vi "VelocityRamp_r0.vi"(10 "Current Velocity (RPS)":dbl, 11 "Input Velocity (RPS)":dbl) -> (3 "Output Velocity (RPS)":dbl)   [LabVIEW 2015]
panel:
  in  "Step Delay (ms)":u32
  out "Waveform Chart":dbl(graph)
  in  "Step Size":dbl format="%#_13g"
  in  "Threshold":dbl format="%#_13g"
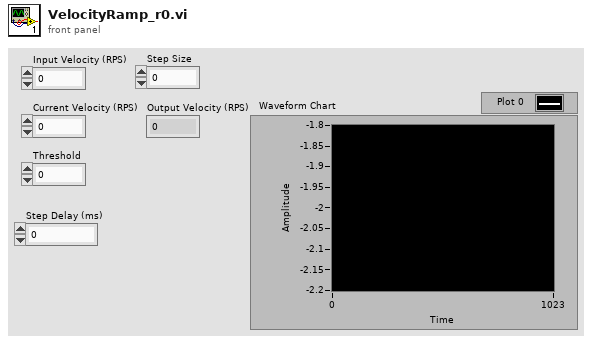
[diagram p1: front panel]
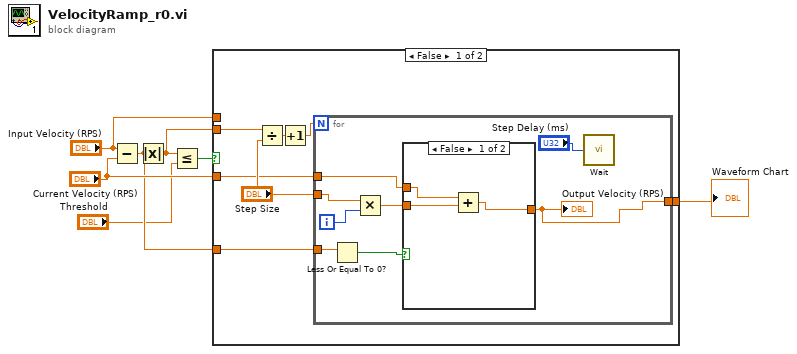
[diagram p0: block diagram]
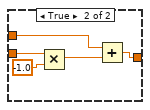
[diagram p2: hidden frame]
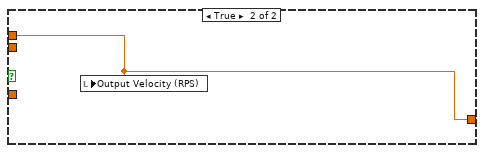
[diagram p3: hidden frame]
diagram:
  n1 = Subtract(x="Input Velocity (RPS)", y="Current Velocity (RPS)") -> (x-y=w4:dbl)
  n2 = Absolute Value(x=w4) -> (abs(x)=w3:dbl)
  n3 = Less Or Equal?(x=w3, y="Threshold") -> (x <= y?=w2:bool)
  n4 = case shown="False" w2 {
    tunnel: "Input Velocity (RPS)" -> [_ w31]
    tunnel: w3 -> [w14 _]
    tunnel: w4 -> [w12 _]
    tunnel: [w11 w31] -> w5
    tunnel: "Current Velocity (RPS)" -> [w8 _]
    frame False {
      n5 = Divide(x=w14, y="Step Size") -> (x/y=w10:dbl)
      n6 = Increment(x=w10) -> (x+1=w9:dbl)
      n7 = for {
        N: w9 -> [_]
        tunnel: "Step Size" -> [w22]
        tunnel: w12 -> [w20]
        tunnel: [w17] -> w11
        tunnel: w8 -> [w16]
        i -> [w21]
        n8 = Less Or Equal To 0?(x=w20) -> (x <= 0?=w19:bool)
        n9 = Multiply(x=w22, y=w21) -> (x*y=w18:dbl)
        n10 = case shown="False" w19 {
          tunnel: w18 -> [w24 w30]
          tunnel: w16 -> [w25 w28]
          tunnel: [w23 w26] -> w17
          frame False {
            n11 = Add(x=w25, y=w24) -> (x+y=w23:dbl)
          }
          frame True {
            n12 = Multiply(x=w30, y=-1.0) -> (x*y=w27:dbl)
            n13 = Add(x=w28, y=w27) -> (x+y=w26:dbl)
          }
        }
        "Output Velocity (RPS)" <- w17
        n14 = call "Wait"("Count(mSec)"="Step Delay (ms)") -> ()  [unwired: 1 out]
      }
    }
    frame True {
      n15 = local write "Output Velocity (RPS)"(w31) -> ()
    }
  }
  "Waveform Chart" <- w5
